vi "niDTS BT INSTR TX Initiate.vi"(8 "error in (no error)":errorcluster, 9 "Result Instance":i32, 10 "Driver Instance":i32, 11 "niDTS BT INSTR TX in":refnum<class "niDTS BT INSTR TX.lvclass">) -> (0 "error out":errorcluster, 3 "niDTS BT INSTR TX out":refnum<class "niDTS BT INSTR TX.lvclass">)   [LabVIEW 2015, in "niDTS BT.lvlib" / "niDTS BT INSTR TX.lvclass"]
uses:
  niDTS BT INSTR TX.lvclass
  niDTS BT INSTR TX.lvclass/niDTS BT INSTR TX.ctl
  RiviInstDriver/niRfsaBT/Objects/niRfsaBt.lvclass
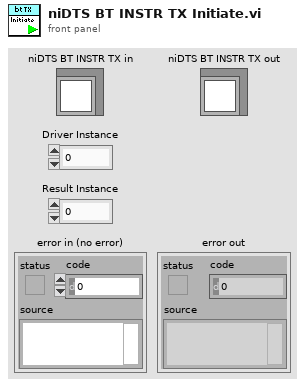
[diagram p1: front panel]
types:
  T1 = typedef "niRfsaBT.lvclass/niRfsaBT INC Handle.ctl" = refnum<data-value>
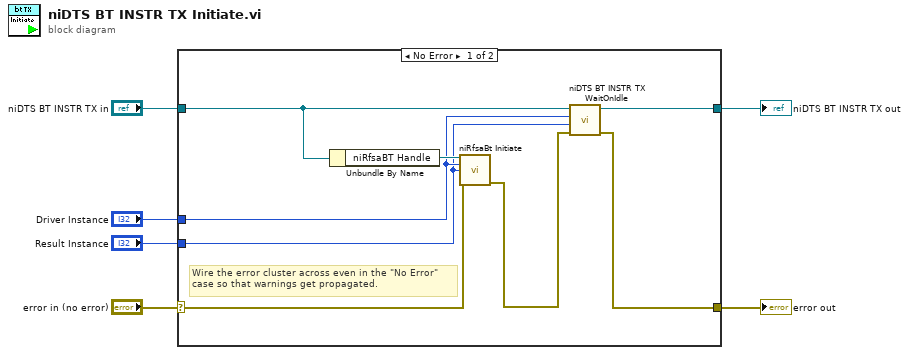
[diagram p0: block diagram]
diagram:
  n1 = case shown="No Error" "error in (no error)" {
    selector: "error in (no error)" -> [w13 w16]
    tunnel: [w9 w16] -> w5
    tunnel: [w11 w15] -> w3
    tunnel: "niDTS BT INSTR TX in" -> [w12 w15]
    tunnel: "Driver Instance" -> [w8 _]
    tunnel: "Result Instance" -> [w7 _]
    frame No Error {
      # "Wire the error cluster across even in the \"No Error\"\ncase so that warnings get propagated."
      n2 = Unbundle By Name(w12) -> ("niRfsaBT Handle"=w14:T1)
      n3 = call "niRfsaBt Initiate.vi"("InstDriver Handle in"=w14, "Driver Instance"=w8, "Result Instance"=w7, "error in (no error)"=w13) -> ("error out"=w10:errorcluster)  [unwired: 10 in, 1 out]
      n4 = call-dynamic "niDTS BT INSTR TX WaitOnIdle.vi"("error in (no error)"=w10, "Result Instance"=w7, "Driver Instance"=w8, "niDTS BT INSTR TX in"=w12) -> ("error out"=w9:errorcluster, "niDTS BT INSTR TX out"=w11:refnum<class "niDTS BT INSTR TX.lvclass">)  [unwired: 6 in]
    }
    frame Error {
    }
  }
  "error out" <- w5
  "niDTS BT INSTR TX out" <- w3
